vi "Generate Silence.vi"(9 "Duration (1 second)":dbl=1.0) -> (3 "Silence out":refnum<class "Silence.lvclass">)   [LabVIEW 2017, in "Silence.lvclass"]
uses:
  Silence.lvclass
  Silence.lvclass/Silence.ctl
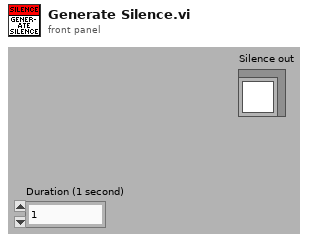
[diagram p1: front panel]
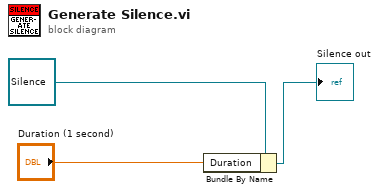
[diagram p0: block diagram]
diagram:
  n1 = Bundle By Name(cluster=refnum<class "Silence.lvclass"> refnum ("Single Tone in"), "Duration"="Duration (1 second)") -> (→"Silence out":refnum<class "Silence.lvclass">)
